vi "SetTrigEdge.vi"(8 "TrigEdge":u8(ring)=1 items=["下降沿", "上升沿"], 11 "错误输入（无错误）":errorcluster) -> (3 "错误输出":errorcluster)   [LabVIEW 2016]
uses:
  PLC-Lab/lib/gusb.dll
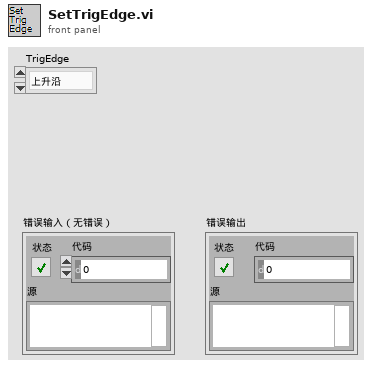
[diagram p1: front panel]
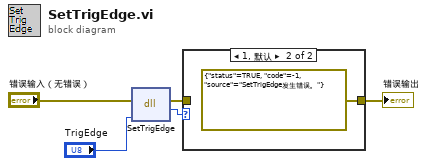
[diagram p0: block diagram]
diagram:
  n1 = dll-call lib="E:/Camproject/2018/2018.1Labview/PLC-Lab/lib/gusb.dll" fn="SetTrigEdge"(error in="错误输入（无错误）", "trigedge"="TrigEdge") -> (error out=w4:errorcluster, "返回类型"=w2:i32)  [unwired: 3 in, 1 out]
  n2 = case shown="1, 默认" w2 {
    tunnel: w4 -> [w6 _]
    tunnel: [w6 errorcluster {"status"=TRUE, "code"=-1, "source"="SetTrigEdge发生错误。"} ("错误常量")] -> w3
    frame 0 {
    }
    frame 1, Default {
    }
  }
  "错误输出" <- w3
